vi "svx_Colormap Response User Shortcut Selection.vi"(6 "Action In":T4, 7 "Data In":T3 {"Y scale"."multiplier" format="%.2f"; "Y scale"."offset" format="%.2f"; "X scale"."multiplier" format="%.2f"; "X scale"."offset" format="%.2f"; "spectral map" format="%.2f"}, 8 "Color Map in":refnum<vi>, 9 "Refnum":refnum<vi>, 10 "ItemTag":string, 11 "State in":T1={"RefQueue"=refnum, "Properties/Undo"=refnum, "Bound"={"Width"=0, "Height"=0}, "Plot Area:Colors"={"FG Color"=11776947, "BG Color"=0}, "scale legend visible?"=FALSE, "graph palette visible?"=FALSE, "cursor palette visible?"=FALSE, "Ignore Array"=TRUE, "Smooth Update"=FALSE, "Z Scale"={"Z Scale.Scale Fit"=2, "Z Scale.Name Label.Text"="Amplitude", "Z Scale.Interpolate Color"=TRUE, "Visible"=TRUE, "Label Visible"=TRUE, "format string"="%#.2g", "Z Scale.Range"={"Minimum"=0.0, "Maximum"=500.0}}, "X Scale"={"X Scale.Scale Fit"=2, "X Scale.Offset and Multiplier"={"Offset"=0.0, "Multiplier"=1.0}, "X Scale.Name Label.Text"="Time", "X Scale.Range"={"Minimum"=0.0, "Maximum"=10.0}, "Visible"=TRUE, "Label Visible"=TRUE, "format string"="%#.2g"}, "Y Scale"={"Y Scale.Scale Fit"=2, "Y Scale.Offset and Multiplier"={"Offset"=0.0, "Multiplier"=1.0}, "Y Scale.Name Label.Text"="Frequency", "Y Scale.Range"={"Minimum"=0.0, "Maximum"=500.0}, "Visible"=TRUE, "Label Visible"=TRUE, "format string"="%#.2g"}, "Annotation List"=[], "Cursor List"=[], "Display Frequency Lines"=TRUE, "Display Order Lines"=TRUE, "Display Order text"=TRUE, "Display Frequency text"=TRUE, "Order Lineproperty"={"Line"={"Width"=1, "Style"=enum."Dash"}, "color"=0}, "Order Textproperty"={"Test size"=11, "color"=16777222, "background"=16777216}, "Orders"=[], "Frequency"=[], "Frequency Lineproperty"={"Line"={"Width"=1, "Style"=enum."Dash"}, "color"=0}, "Frequency Textproperty"={"Test size"=11, "color"=16777222, "background"=16777216}, "Display Order from Cursor"=FALSE, "Display Freq from Cursor"=FALSE, "Active Cursor"=0, "Selected Cursors"=[], "Cursor Move"=refnum, "Scale Range Change"=refnum}) -> (0 "Events":T2[](array[typedef]), 3 "State out":T1={"RefQueue"=refnum, "Properties/Undo"=refnum, "Bound"={"Width"=0, "Height"=0}, "Plot Area:Colors"={"FG Color"=11776947, "BG Color"=0}, "scale legend visible?"=FALSE, "graph palette visible?"=FALSE, "cursor palette visible?"=FALSE, "Ignore Array"=TRUE, "Smooth Update"=FALSE, "Z Scale"={"Z Scale.Scale Fit"=2, "Z Scale.Name Label.Text"="Amplitude", "Z Scale.Interpolate Color"=TRUE, "Visible"=TRUE, "Label Visible"=TRUE, "format string"="%#.2g", "Z Scale.Range"={"Minimum"=0.0, "Maximum"=500.0}}, "X Scale"={"X Scale.Scale Fit"=2, "X Scale.Offset and Multiplier"={"Offset"=0.0, "Multiplier"=1.0}, "X Scale.Name Label.Text"="Time", "X Scale.Range"={"Minimum"=0.0, "Maximum"=10.0}, "Visible"=TRUE, "Label Visible"=TRUE, "format string"="%#.2g"}, "Y Scale"={"Y Scale.Scale Fit"=2, "Y Scale.Offset and Multiplier"={"Offset"=0.0, "Multiplier"=1.0}, "Y Scale.Name Label.Text"="Frequency", "Y Scale.Range"={"Minimum"=0.0, "Maximum"=500.0}, "Visible"=TRUE, "Label Visible"=TRUE, "format string"="%#.2g"}, "Annotation List"=[], "Cursor List"=[], "Display Frequency Lines"=TRUE, "Display Order Lines"=TRUE, "Display Order text"=TRUE, "Display Frequency text"=TRUE, "Order Lineproperty"={"Line"={"Width"=1, "Style"=enum."Dash"}, "color"=0}, "Order Textproperty"={"Test size"=11, "color"=16777222, "background"=16777216}, "Orders"=[], "Frequency"=[], "Frequency Lineproperty"={"Line"={"Width"=1, "Style"=enum."Dash"}, "color"=0}, "Frequency Textproperty"={"Test size"=11, "color"=16777222, "background"=16777216}, "Display Order from Cursor"=FALSE, "Display Freq from Cursor"=FALSE, "Active Cursor"=0, "Selected Cursors"=[], "Cursor Move"=refnum, "Scale Range Change"=refnum}, 4 "Action":T4)   [LabVIEW 2017, in "SVX Colormap.xctl"]
uses:
  <vilib>/addons/_XControls/Colormap/SVX Colormap.xctl
  <vilib>/_xctls/Action.ctl
  <vilib>/addons/_XControls/Colormap/subVIs/svx_Colormap Data.ctl
  <vilib>/addons/_XControls/Colormap/TypeDef/svx_Colormap_Event.ctl
  <vilib>/addons/_XControls/Colormap/subVIs/svx_Colormap State.ctl
  <vilib>/addons/_XControls/Colormap/TypeDef/svx_Colormap_InnerState.ctl
  <vilib>/_xctls/XControlSupport.lvlib
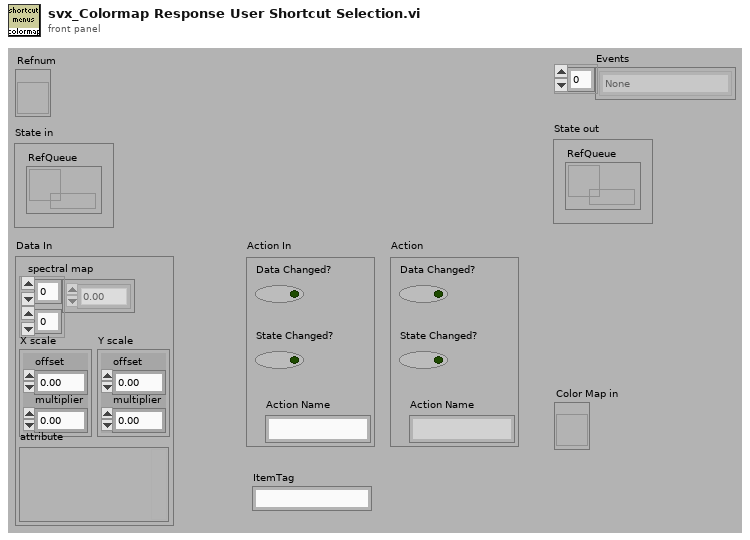
[diagram p1: front panel]
types:
  T1 = typedef "SVX Colormap.xctl/svx_Colormap State.ctl" = cluster{"RefQueue":refnum<queue>, "Properties/Undo":refnum<queue>, "Bound":cluster{"Width":u32, "Height":u32}, "Plot Area:Colors":cluster{"FG Color":u32, "BG Color":u32}, "scale legend visible?":bool, "graph palette visible?":bool, "cursor palette visible?":bool, "Ignore Array":bool, "Smooth Update":bool, "Z Scale":cluster{"Z Scale.Scale Fit":u8, "Z Scale.Name Label.Text":string, "Z Scale.Interpolate Color":bool, "Visible":bool, "Label Visible":bool, "format string":string, "Z Scale.Range":cluster{"Minimum":dbl, "Maximum":dbl}}, "X Scale":cluster{"X Scale.Scale Fit":u8, "X Scale.Offset and Multiplier":cluster{"Offset":dbl, "Multiplier":dbl}, "X Scale.Name Label.Text":string, "X Scale.Range":cluster{"Minimum":dbl, "Maximum":dbl}, "Visible":bool, "Label Visible":bool, "format string":string}, "Y Scale":cluster{"Y Scale.Scale Fit":u8, "Y Scale.Offset and Multiplier":cluster{"Offset":dbl, "Multiplier":dbl}, "Y Scale.Name Label.Text":string, "Y Scale.Range":cluster{"Minimum":dbl, "Maximum":dbl}, "Visible":bool, "Label Visible":bool, "format string":string}, "Annotation List":cluster{"Name":string, "Color":u32, "Style":u8, "Point Style":u8, "Name Visible":bool, "Allow Drag":bool, "Annotation Mode":u32, "Plot":i32, "Index":i32, "Position":cluster{"X":dbl, "Y":dbl}, "X Scale":u32, "Y Scale":u32, "Show Arrow":bool, "Lock Name":bool, "Plot Area":i32, "Label Offset":cluster{"X":dbl, "Y":dbl}}[], "Cursor List":cluster{"Name":string, "Color":u32, "Style":u8, "Point Style":u8, "Name Visible":bool, "Allow Drag":bool, "Cursor Mode":u32, "Plot":i32, "Index":i32, "Position":cluster{"X":dbl, "Y":dbl}, "X Scale":u32, "Y Scale":u32, "Watch Plots":i32[], "Watch All Plots":bool, "Plot Area":i32, "Label Offset":cluster{"X":dbl, "Y":dbl}}[], "Display Frequency Lines":bool, "Display Order Lines":bool, "Display Order text":bool, "Display Frequency text":bool, "Order Lineproperty":cluster{"Line":cluster{"Width":u16, "Style":enum32{"Solid", "Dash", "Dot", "DashDot", "DashDotDot"}}, "color":u32}, "Order Textproperty":cluster{"Test size":i16, "color":u32, "background":u32}, "Orders":dbl[], "Frequency":dbl[], "Frequency Lineproperty":cluster{"Line":cluster{"Width":u16, "Style":enum32{"Solid", "Dash", "Dot", "DashDot", "DashDotDot"}}, "color":u32}, "Frequency Textproperty":cluster{"Test size":i16, "color":u32, "background":u32}, "Display Order from Cursor":bool, "Display Freq from Cursor":bool, "Active Cursor":u32, "Selected Cursors":u32[], "Cursor Move":refnum<user-event>, "Scale Range Change":refnum<user-event>}
  T2 = typedef "SVX Colormap.xctl/svx_Colormap_Event.ctl" = enum16{"None", "[Axis] X Range", "[Axis] Y Range", "[Axis] Z Range", "[Axis] Range", "[Axis] X FString", "[Axis] Y FString", "[Axis] Z FString", "[Axis] X Name", "[Axis] X ScaleVis", "[Axis] X NameVis", "[Axis] Y Name", "[Axis] Y ScaleVis", "[Axis] Y NameVis", "[Axis] Z Name", "[Axis] Z ScaleVis", "[Axis] Z NameVis", "[Image] Line", "[Axis] Z Interp", "[Data] Update", "[Layout] Resize", "[ColorTable] Ignore Array", "[Legend] ScaleVis", "[Legend] GPVis", "[Legend] CPVis", "[Smooth] Update", "[Cursor] Update", "[Plot Area] Colors", "[Size] Minimum", "[Annotation] Update", "[Properties Dialog]", "[Axis] Autoscale X", "[Axis] Autoscale Y", "[Axis] Autoscale Z"}
  T3 = typedef "SVX Colormap.xctl/svx_Colormap Data.ctl" = cluster{"spectral map":dbl[][], "X scale":cluster{"offset":dbl, "multiplier":dbl}, "Y scale":cluster{"offset":dbl, "multiplier":dbl}, "attribute":variant}
  T4 = typedef "XControlSupport.lvlib/Action.ctl" = cluster{"Data Changed?":bool, "State Changed?":bool, "Action Name":string}
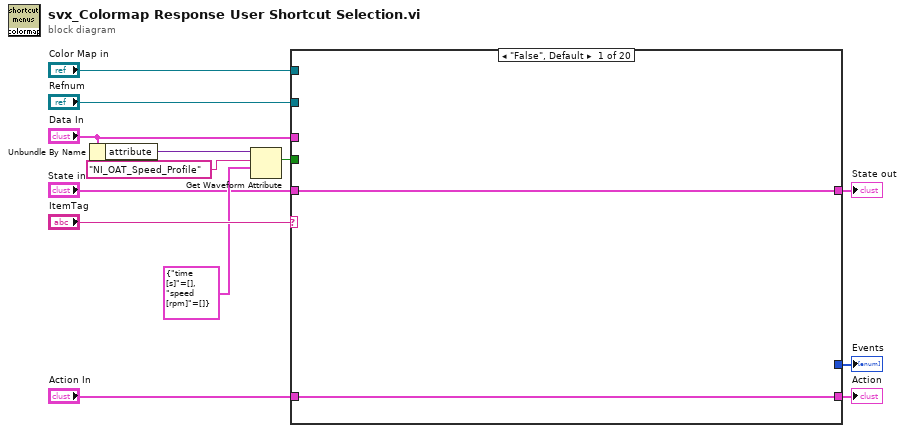
[diagram p0: block diagram]
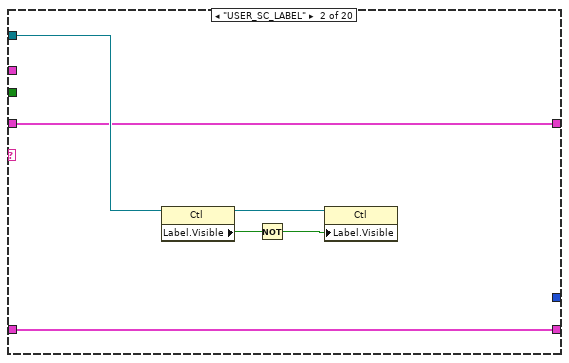
[diagram p2: hidden frame]
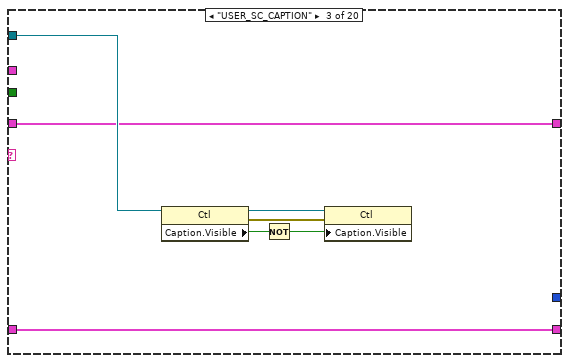
[diagram p3: hidden frame]
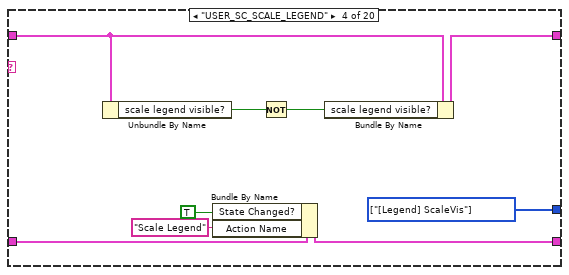
[diagram p4: hidden frame]
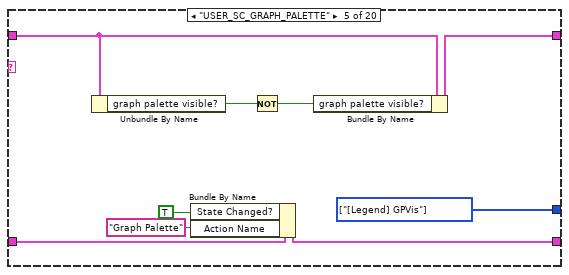
[diagram p5: hidden frame]
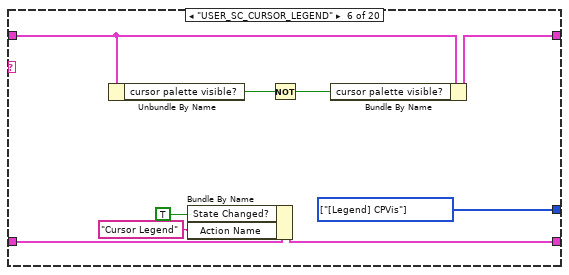
[diagram p6: hidden frame]
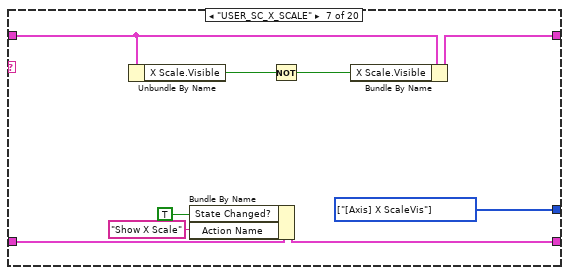
[diagram p7: hidden frame]
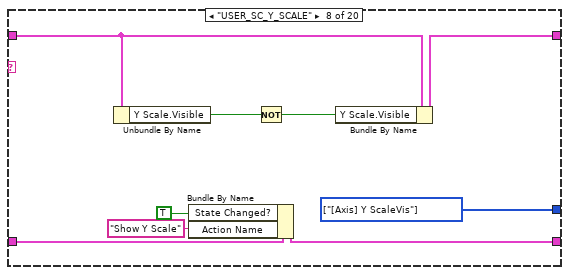
[diagram p8: hidden frame]
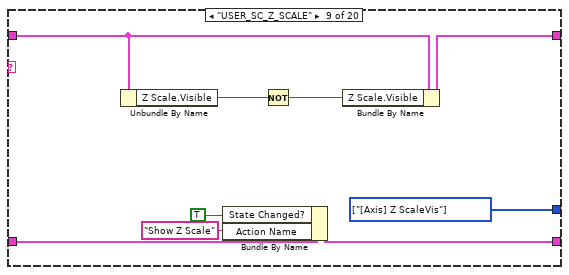
[diagram p9: hidden frame]
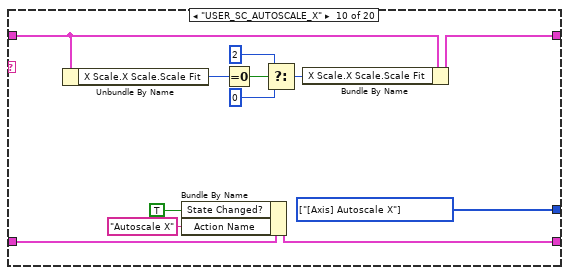
[diagram p10: hidden frame]
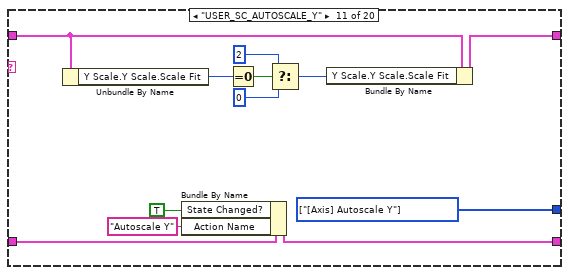
[diagram p11: hidden frame]
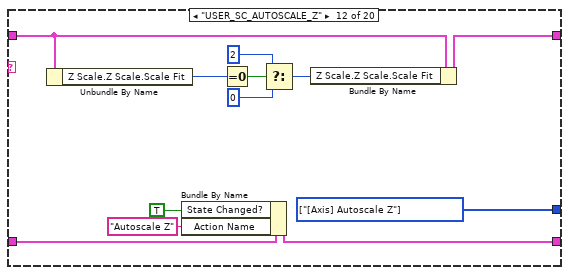
[diagram p12: hidden frame]
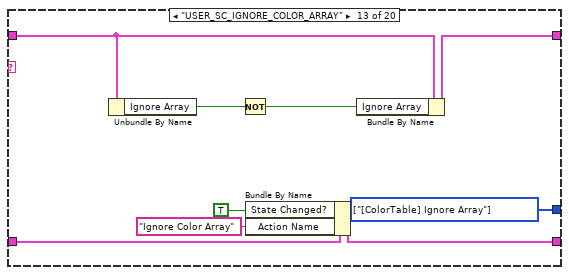
[diagram p13: hidden frame]
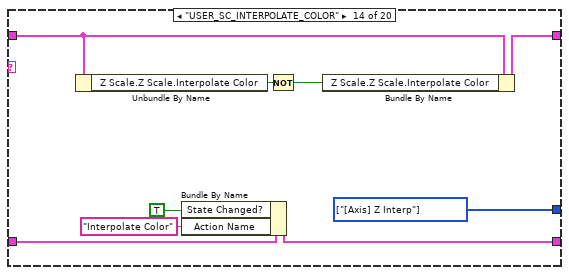
[diagram p14: hidden frame]
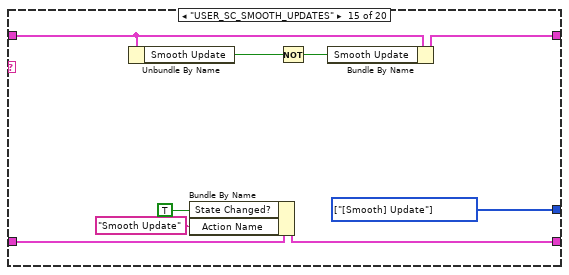
[diagram p15: hidden frame]
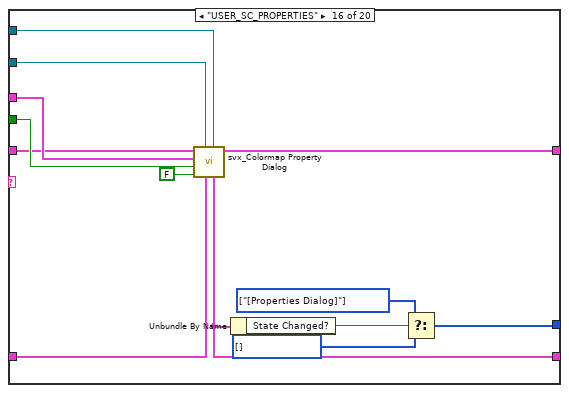
[diagram p16: hidden frame]
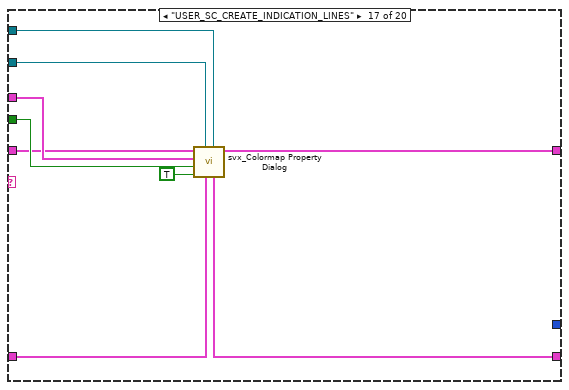
[diagram p17: hidden frame]
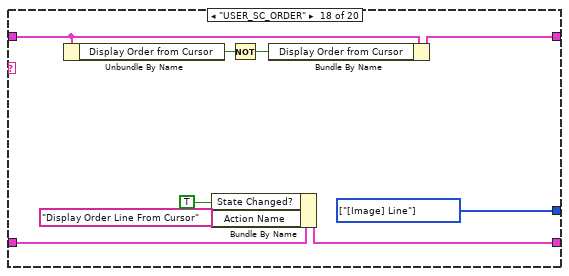
[diagram p18: hidden frame]
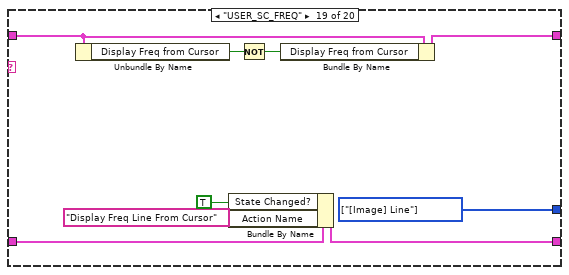
[diagram p19: hidden frame]
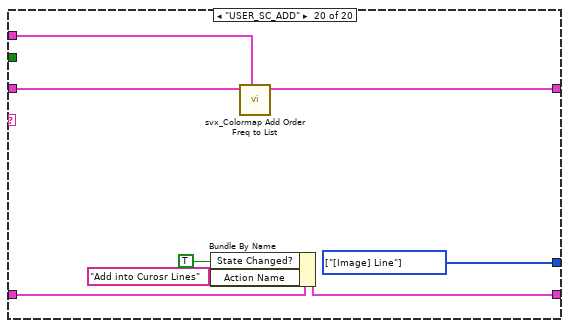
[diagram p20: hidden frame]
diagram:
  n1 = Unbundle By Name("Data In") -> ("attribute"=w9:variant)
  n2 = Get Waveform Attribute(5:cluster{"time [s]":dbl[], "speed [rpm]":dbl[]} {"time [s]"=[], "speed [rpm]"=[]} ("speed profile"), 6:"NI_OAT_Speed_Profile" ("name"), 7:w9) -> (2:w6:bool)  [unwired: 1 in, 3 out]
  n3 = case shown="\"False\", Default" "ItemTag" {
    tunnel: "Refnum" -> [_ w18 w24 _ _ _ _ _ _ _ _ _ _ _ _ w156 w164 _ _ _]
    tunnel: "Action In" -> [w15 w16 w22 w37 w46 w55 w62 w71 w80 w94 w106 w118 w127 w136 w145 w158 w166 w171 w178 w190]
    tunnel: [w15 w16 w22 w36 w45 w54 w61 w70 w79 w93 w105 w117 w126 w135 w144 w150 w167 w170 w179 w189] -> w11
    tunnel: "Color Map in" -> [_ _ _ _ _ _ _ _ _ _ _ _ _ _ _ w155 w163 _ _ _]
    tunnel: "State in" -> [w14 w17 w23 w31 w40 w49 w58 w67 w76 w89 w101 w113 w121 w131 w139 w152 w160 w176 w181 w191]
    tunnel: [w14 w17 w23 w33 w39 w48 w57 w66 w75 w90 w102 w114 w120 w132 w141 w157 w165 w175 w180 w193] -> w1
    tunnel: [_ _ _ w32 w38 w47 w56 w65 w74 w88 w100 w112 w119 w128 w137 w148 _ w168 w177 w186] -> w3
    tunnel: w6 -> [_ _ _ _ _ _ _ _ _ _ _ _ _ _ _ w153 w161 _ _ _]
    tunnel: "Data In" -> [_ _ _ _ _ _ _ _ _ _ _ _ _ _ _ w154 w162 _ _ w192]
    frame "False", Default {
    }
    frame "USER_SC_LABEL" {
      n4 = property class="Ctl"(reference=w18) -> (reference out=w21:refnum<vi>, "Label.Visible"=w20:bool)  [unwired: 1 in, 1 out]
      n5 = Not(x=w20) -> (.not. x?=w19:bool)
      n6 = property class="Ctl"(reference=w21, "Label.Visible"=w19) -> ()  [unwired: 1 in, 2 out]
    }
    frame "USER_SC_CAPTION" {
      n7 = property class="Ctl"(reference=w24) -> (reference out=w28:refnum<vi>, error out=w27:errorcluster, "Caption.Visible"=w26:bool)  [unwired: 1 in]
      n8 = Not(x=w26) -> (.not. x?=w25:bool)
      n9 = property class="Ctl"(reference=w28, error in=w27, "Caption.Visible"=w25) -> ()  [unwired: 2 out]
    }
    frame "USER_SC_SCALE_LEGEND" {
      w32 = T2[] [enum."[Legend] ScaleVis"] items=["None", "[Axis] X Range", "[Axis] Y Range", "[Axis] Z Range", "[Axis] Range", "[Axis] X FString", "[Axis] Y FString", "[Axis] Z FString", "[Axis] X Name", "[Axis] X ScaleVis", "[Axis] X NameVis", "[Axis] Y Name", "[Axis] Y ScaleVis", "[Axis] Y NameVis", "[Axis] Z Name", "[Axis] Z ScaleVis", "[Axis] Z NameVis", "[Image] Line", "[Axis] Z Interp", "[Data] Update", "[Layout] Resize", "[ColorTable] Ignore Array", "[Legend] ScaleVis", "[Legend] GPVis", "[Legend] CPVis", "[Smooth] Update", "[Cursor] Update", "[Plot Area] Colors", "[Size] Minimum", "[Annotation] Update", "[Properties Dialog]", "[Axis] Autoscale X", "[Axis] Autoscale Y", "[Axis] Autoscale Z"]
      n10 = Unbundle By Name(w31) -> ("scale legend visible?"=w30:bool)
      n11 = Bundle By Name(cluster=w37, "State Changed?"=TRUE, "Action Name"="Scale Legend") -> (w36:T4)
      n12 = Not(x=w30) -> (.not. x?=w29:bool)
      n13 = Bundle By Name(cluster=w31, "scale legend visible?"=w29) -> (w33:T1)
    }
    frame "USER_SC_GRAPH_PALETTE" {
      w38 = T2[] [enum."[Legend] GPVis"] items=["None", "[Axis] X Range", "[Axis] Y Range", "[Axis] Z Range", "[Axis] Range", "[Axis] X FString", "[Axis] Y FString", "[Axis] Z FString", "[Axis] X Name", "[Axis] X ScaleVis", "[Axis] X NameVis", "[Axis] Y Name", "[Axis] Y ScaleVis", "[Axis] Y NameVis", "[Axis] Z Name", "[Axis] Z ScaleVis", "[Axis] Z NameVis", "[Image] Line", "[Axis] Z Interp", "[Data] Update", "[Layout] Resize", "[ColorTable] Ignore Array", "[Legend] ScaleVis", "[Legend] GPVis", "[Legend] CPVis", "[Smooth] Update", "[Cursor] Update", "[Plot Area] Colors", "[Size] Minimum", "[Annotation] Update", "[Properties Dialog]", "[Axis] Autoscale X", "[Axis] Autoscale Y", "[Axis] Autoscale Z"]
      n14 = Unbundle By Name(w40) -> ("graph palette visible?"=w42:bool)
      n15 = Bundle By Name(cluster=w46, "State Changed?"=TRUE, "Action Name"="Graph Palette") -> (w45:T4)
      n16 = Not(x=w42) -> (.not. x?=w41:bool)
      n17 = Bundle By Name(cluster=w40, "graph palette visible?"=w41) -> (w39:T1)
    }
    frame "USER_SC_CURSOR_LEGEND" {
      w47 = T2[] [enum."[Legend] CPVis"] items=["None", "[Axis] X Range", "[Axis] Y Range", "[Axis] Z Range", "[Axis] Range", "[Axis] X FString", "[Axis] Y FString", "[Axis] Z FString", "[Axis] X Name", "[Axis] X ScaleVis", "[Axis] X NameVis", "[Axis] Y Name", "[Axis] Y ScaleVis", "[Axis] Y NameVis", "[Axis] Z Name", "[Axis] Z ScaleVis", "[Axis] Z NameVis", "[Image] Line", "[Axis] Z Interp", "[Data] Update", "[Layout] Resize", "[ColorTable] Ignore Array", "[Legend] ScaleVis", "[Legend] GPVis", "[Legend] CPVis", "[Smooth] Update", "[Cursor] Update", "[Plot Area] Colors", "[Size] Minimum", "[Annotation] Update", "[Properties Dialog]", "[Axis] Autoscale X", "[Axis] Autoscale Y", "[Axis] Autoscale Z"]
      n18 = Unbundle By Name(w49) -> ("cursor palette visible?"=w51:bool)
      n19 = Bundle By Name(cluster=w55, "State Changed?"=TRUE, "Action Name"="Cursor Legend") -> (w54:T4)
      n20 = Not(x=w51) -> (.not. x?=w50:bool)
      n21 = Bundle By Name(cluster=w49, "cursor palette visible?"=w50) -> (w48:T1)
    }
    frame "USER_SC_X_SCALE" {
      w56 = T2[] [enum."[Axis] X ScaleVis"] items=["None", "[Axis] X Range", "[Axis] Y Range", "[Axis] Z Range", "[Axis] Range", "[Axis] X FString", "[Axis] Y FString", "[Axis] Z FString", "[Axis] X Name", "[Axis] X ScaleVis", "[Axis] X NameVis", "[Axis] Y Name", "[Axis] Y ScaleVis", "[Axis] Y NameVis", "[Axis] Z Name", "[Axis] Z ScaleVis", "[Axis] Z NameVis", "[Image] Line", "[Axis] Z Interp", "[Data] Update", "[Layout] Resize", "[ColorTable] Ignore Array", "[Legend] ScaleVis", "[Legend] GPVis", "[Legend] CPVis", "[Smooth] Update", "[Cursor] Update", "[Plot Area] Colors", "[Size] Minimum", "[Annotation] Update", "[Properties Dialog]", "[Axis] Autoscale X", "[Axis] Autoscale Y", "[Axis] Autoscale Z"]
      n22 = Unbundle By Name(w58) -> ("X Scale.Visible"=w60:bool)
      n23 = Bundle By Name(cluster=w62, "State Changed?"=TRUE, "Action Name"="Show X Scale") -> (w61:T4)
      n24 = Not(x=w60) -> (.not. x?=w59:bool)
      n25 = Bundle By Name(cluster=w58, "X Scale.Visible"=w59) -> (w57:T1)
    }
    frame "USER_SC_Y_SCALE" {
      w65 = T2[] [enum."[Axis] Y ScaleVis"] items=["None", "[Axis] X Range", "[Axis] Y Range", "[Axis] Z Range", "[Axis] Range", "[Axis] X FString", "[Axis] Y FString", "[Axis] Z FString", "[Axis] X Name", "[Axis] X ScaleVis", "[Axis] X NameVis", "[Axis] Y Name", "[Axis] Y ScaleVis", "[Axis] Y NameVis", "[Axis] Z Name", "[Axis] Z ScaleVis", "[Axis] Z NameVis", "[Image] Line", "[Axis] Z Interp", "[Data] Update", "[Layout] Resize", "[ColorTable] Ignore Array", "[Legend] ScaleVis", "[Legend] GPVis", "[Legend] CPVis", "[Smooth] Update", "[Cursor] Update", "[Plot Area] Colors", "[Size] Minimum", "[Annotation] Update", "[Properties Dialog]", "[Axis] Autoscale X", "[Axis] Autoscale Y", "[Axis] Autoscale Z"]
      n26 = Unbundle By Name(w67) -> ("Y Scale.Visible"=w69:bool)
      n27 = Bundle By Name(cluster=w71, "State Changed?"=TRUE, "Action Name"="Show Y Scale") -> (w70:T4)
      n28 = Not(x=w69) -> (.not. x?=w68:bool)
      n29 = Bundle By Name(cluster=w67, "Y Scale.Visible"=w68) -> (w66:T1)
    }
    frame "USER_SC_Z_SCALE" {
      w74 = T2[] [enum."[Axis] Z ScaleVis"] items=["None", "[Axis] X Range", "[Axis] Y Range", "[Axis] Z Range", "[Axis] Range", "[Axis] X FString", "[Axis] Y FString", "[Axis] Z FString", "[Axis] X Name", "[Axis] X ScaleVis", "[Axis] X NameVis", "[Axis] Y Name", "[Axis] Y ScaleVis", "[Axis] Y NameVis", "[Axis] Z Name", "[Axis] Z ScaleVis", "[Axis] Z NameVis", "[Image] Line", "[Axis] Z Interp", "[Data] Update", "[Layout] Resize", "[ColorTable] Ignore Array", "[Legend] ScaleVis", "[Legend] GPVis", "[Legend] CPVis", "[Smooth] Update", "[Cursor] Update", "[Plot Area] Colors", "[Size] Minimum", "[Annotation] Update", "[Properties Dialog]", "[Axis] Autoscale X", "[Axis] Autoscale Y", "[Axis] Autoscale Z"]
      n30 = Unbundle By Name(w76) -> ("Z Scale.Visible"=w78:bool)
      n31 = Bundle By Name(cluster=w80, "State Changed?"=TRUE, "Action Name"="Show Z Scale") -> (w79:T4)
      n32 = Not(x=w78) -> (.not. x?=w77:bool)
      n33 = Bundle By Name(cluster=w76, "Z Scale.Visible"=w77) -> (w75:T1)
    }
    frame "USER_SC_AUTOSCALE_X" {
      w88 = T2[] [enum."[Axis] Autoscale X"] items=["None", "[Axis] X Range", "[Axis] Y Range", "[Axis] Z Range", "[Axis] Range", "[Axis] X FString", "[Axis] Y FString", "[Axis] Z FString", "[Axis] X Name", "[Axis] X ScaleVis", "[Axis] X NameVis", "[Axis] Y Name", "[Axis] Y ScaleVis", "[Axis] Y NameVis", "[Axis] Z Name", "[Axis] Z ScaleVis", "[Axis] Z NameVis", "[Image] Line", "[Axis] Z Interp", "[Data] Update", "[Layout] Resize", "[ColorTable] Ignore Array", "[Legend] ScaleVis", "[Legend] GPVis", "[Legend] CPVis", "[Smooth] Update", "[Cursor] Update", "[Plot Area] Colors", "[Size] Minimum", "[Annotation] Update", "[Properties Dialog]", "[Axis] Autoscale X", "[Axis] Autoscale Y", "[Axis] Autoscale Z"]
      n34 = Unbundle By Name(w89) -> ("X Scale.X Scale.Scale Fit"=w87:u8)
      n35 = Bundle By Name(cluster=w94, "State Changed?"=TRUE, "Action Name"="Autoscale X") -> (w93:T4)
      n36 = Equal To 0?(x=w87) -> (x = 0?=w86:bool)
      n37 = Select(t=u8 2 ("X Scale.X Scale.Scale Fit"), s=w86, f=u8 0 ("X Scale.X Scale.Scale Fit")) -> (s? t:f=w83:u8)
      n38 = Bundle By Name(cluster=w89, "X Scale.X Scale.Scale Fit"=w83) -> (w90:T1)
    }
    frame "USER_SC_AUTOSCALE_Y" {
      w100 = T2[] [enum."[Axis] Autoscale Y"] items=["None", "[Axis] X Range", "[Axis] Y Range", "[Axis] Z Range", "[Axis] Range", "[Axis] X FString", "[Axis] Y FString", "[Axis] Z FString", "[Axis] X Name", "[Axis] X ScaleVis", "[Axis] X NameVis", "[Axis] Y Name", "[Axis] Y ScaleVis", "[Axis] Y NameVis", "[Axis] Z Name", "[Axis] Z ScaleVis", "[Axis] Z NameVis", "[Image] Line", "[Axis] Z Interp", "[Data] Update", "[Layout] Resize", "[ColorTable] Ignore Array", "[Legend] ScaleVis", "[Legend] GPVis", "[Legend] CPVis", "[Smooth] Update", "[Cursor] Update", "[Plot Area] Colors", "[Size] Minimum", "[Annotation] Update", "[Properties Dialog]", "[Axis] Autoscale X", "[Axis] Autoscale Y", "[Axis] Autoscale Z"]
      n39 = Unbundle By Name(w101) -> ("Y Scale.Y Scale.Scale Fit"=w96:u8)
      n40 = Bundle By Name(cluster=w106, "State Changed?"=TRUE, "Action Name"="Autoscale Y") -> (w105:T4)
      n41 = Equal To 0?(x=w96) -> (x = 0?=w99:bool)
      n42 = Select(t=u8 2 ("X Scale.X Scale.Scale Fit"), s=w99, f=u8 0 ("X Scale.X Scale.Scale Fit")) -> (s? t:f=w95:u8)
      n43 = Bundle By Name(cluster=w101, "Y Scale.Y Scale.Scale Fit"=w95) -> (w102:T1)
    }
    frame "USER_SC_AUTOSCALE_Z" {
      w112 = T2[] [enum."[Axis] Autoscale Z"] items=["None", "[Axis] X Range", "[Axis] Y Range", "[Axis] Z Range", "[Axis] Range", "[Axis] X FString", "[Axis] Y FString", "[Axis] Z FString", "[Axis] X Name", "[Axis] X ScaleVis", "[Axis] X NameVis", "[Axis] Y Name", "[Axis] Y ScaleVis", "[Axis] Y NameVis", "[Axis] Z Name", "[Axis] Z ScaleVis", "[Axis] Z NameVis", "[Image] Line", "[Axis] Z Interp", "[Data] Update", "[Layout] Resize", "[ColorTable] Ignore Array", "[Legend] ScaleVis", "[Legend] GPVis", "[Legend] CPVis", "[Smooth] Update", "[Cursor] Update", "[Plot Area] Colors", "[Size] Minimum", "[Annotation] Update", "[Properties Dialog]", "[Axis] Autoscale X", "[Axis] Autoscale Y", "[Axis] Autoscale Z"]
      n44 = Unbundle By Name(w113) -> ("Z Scale.Z Scale.Scale Fit"=w108:u8)
      n45 = Bundle By Name(cluster=w118, "State Changed?"=TRUE, "Action Name"="Autoscale Z") -> (w117:T4)
      n46 = Equal To 0?(x=w108) -> (x = 0?=w111:bool)
      n47 = Select(t=u8 2 ("X Scale.X Scale.Scale Fit"), s=w111, f=u8 0 ("X Scale.X Scale.Scale Fit")) -> (s? t:f=w107:u8)
      n48 = Bundle By Name(cluster=w113, "Z Scale.Z Scale.Scale Fit"=w107) -> (w114:T1)
    }
    frame "USER_SC_IGNORE_COLOR_ARRAY" {
      w119 = T2[] [enum."[ColorTable] Ignore Array"] items=["None", "[Axis] X Range", "[Axis] Y Range", "[Axis] Z Range", "[Axis] Range", "[Axis] X FString", "[Axis] Y FString", "[Axis] Z FString", "[Axis] X Name", "[Axis] X ScaleVis", "[Axis] X NameVis", "[Axis] Y Name", "[Axis] Y ScaleVis", "[Axis] Y NameVis", "[Axis] Z Name", "[Axis] Z ScaleVis", "[Axis] Z NameVis", "[Image] Line", "[Axis] Z Interp", "[Data] Update", "[Layout] Resize", "[ColorTable] Ignore Array", "[Legend] ScaleVis", "[Legend] GPVis", "[Legend] CPVis", "[Smooth] Update", "[Cursor] Update", "[Plot Area] Colors", "[Size] Minimum", "[Annotation] Update", "[Properties Dialog]", "[Axis] Autoscale X", "[Axis] Autoscale Y", "[Axis] Autoscale Z"]
      n49 = Unbundle By Name(w121) -> ("Ignore Array"=w123:bool)
      n50 = Not(x=w123) -> (.not. x?=w122:bool)
      n51 = Bundle By Name(cluster=w127, "State Changed?"=TRUE, "Action Name"="Ignore Color Array") -> (w126:T4)
      n52 = Bundle By Name(cluster=w121, "Ignore Array"=w122) -> (w120:T1)
    }
    frame "USER_SC_INTERPOLATE_COLOR" {
      w128 = T2[] [enum."[Axis] Z Interp"] items=["None", "[Axis] X Range", "[Axis] Y Range", "[Axis] Z Range", "[Axis] Range", "[Axis] X FString", "[Axis] Y FString", "[Axis] Z FString", "[Axis] X Name", "[Axis] X ScaleVis", "[Axis] X NameVis", "[Axis] Y Name", "[Axis] Y ScaleVis", "[Axis] Y NameVis", "[Axis] Z Name", "[Axis] Z ScaleVis", "[Axis] Z NameVis", "[Image] Line", "[Axis] Z Interp", "[Data] Update", "[Layout] Resize", "[ColorTable] Ignore Array", "[Legend] ScaleVis", "[Legend] GPVis", "[Legend] CPVis", "[Smooth] Update", "[Cursor] Update", "[Plot Area] Colors", "[Size] Minimum", "[Annotation] Update", "[Properties Dialog]", "[Axis] Autoscale X", "[Axis] Autoscale Y", "[Axis] Autoscale Z"]
      n53 = Unbundle By Name(w131) -> ("Z Scale.Z Scale.Interpolate Color"=w130:bool)
      n54 = Bundle By Name(cluster=w136, "State Changed?"=TRUE, "Action Name"="Interpolate Color") -> (w135:T4)
      n55 = Not(x=w130) -> (.not. x?=w129:bool)
      n56 = Bundle By Name(cluster=w131, "Z Scale.Z Scale.Interpolate Color"=w129) -> (w132:T1)
    }
    frame "USER_SC_SMOOTH_UPDATES" {
      w137 = T2[] [enum."[Smooth] Update"] items=["None", "[Axis] X Range", "[Axis] Y Range", "[Axis] Z Range", "[Axis] Range", "[Axis] X FString", "[Axis] Y FString", "[Axis] Z FString", "[Axis] X Name", "[Axis] X ScaleVis", "[Axis] X NameVis", "[Axis] Y Name", "[Axis] Y ScaleVis", "[Axis] Y NameVis", "[Axis] Z Name", "[Axis] Z ScaleVis", "[Axis] Z NameVis", "[Image] Line", "[Axis] Z Interp", "[Data] Update", "[Layout] Resize", "[ColorTable] Ignore Array", "[Legend] ScaleVis", "[Legend] GPVis", "[Legend] CPVis", "[Smooth] Update", "[Cursor] Update", "[Plot Area] Colors", "[Size] Minimum", "[Annotation] Update", "[Properties Dialog]", "[Axis] Autoscale X", "[Axis] Autoscale Y", "[Axis] Autoscale Z"]
      n57 = Unbundle By Name(w139) -> ("Smooth Update"=w140:bool)
      n58 = Bundle By Name(cluster=w145, "State Changed?"=TRUE, "Action Name"="Smooth Update") -> (w144:T4)
      n59 = Not(x=w140) -> (.not. x?=w138:bool)
      n60 = Bundle By Name(cluster=w139, "Smooth Update"=w138) -> (w141:T1)
    }
    frame "USER_SC_PROPERTIES" {
      w146 = T2[] [] items=["None", "[Axis] X Range", "[Axis] Y Range", "[Axis] Z Range", "[Axis] Range", "[Axis] X FString", "[Axis] Y FString", "[Axis] Z FString", "[Axis] X Name", "[Axis] X ScaleVis", "[Axis] X NameVis", "[Axis] Y Name", "[Axis] Y ScaleVis", "[Axis] Y NameVis", "[Axis] Z Name", "[Axis] Z ScaleVis", "[Axis] Z NameVis", "[Image] Line", "[Axis] Z Interp", "[Data] Update", "[Layout] Resize", "[ColorTable] Ignore Array", "[Legend] ScaleVis", "[Legend] GPVis", "[Legend] CPVis", "[Smooth] Update", "[Cursor] Update", "[Plot Area] Colors", "[Size] Minimum", "[Annotation] Update", "[Properties Dialog]", "[Axis] Autoscale X", "[Axis] Autoscale Y", "[Axis] Autoscale Z"] ("f")
      w147 = T2[] [enum."[Properties Dialog]"] items=["None", "[Axis] X Range", "[Axis] Y Range", "[Axis] Z Range", "[Axis] Range", "[Axis] X FString", "[Axis] Y FString", "[Axis] Z FString", "[Axis] X Name", "[Axis] X ScaleVis", "[Axis] X NameVis", "[Axis] Y Name", "[Axis] Y ScaleVis", "[Axis] Y NameVis", "[Axis] Z Name", "[Axis] Z ScaleVis", "[Axis] Z NameVis", "[Image] Line", "[Axis] Z Interp", "[Data] Update", "[Layout] Resize", "[ColorTable] Ignore Array", "[Legend] ScaleVis", "[Legend] GPVis", "[Legend] CPVis", "[Smooth] Update", "[Cursor] Update", "[Plot Area] Colors", "[Size] Minimum", "[Annotation] Update", "[Properties Dialog]", "[Axis] Autoscale X", "[Axis] Autoscale Y", "[Axis] Autoscale Z"]
      n61 = call <vilib>:"svx_Colormap Property Dialog.vi"("Color Map in"=w155, "Action In"=w158, "Refnum"=w156, "Cursor Lines only?"=FALSE, "Found Speed"=w153, "Data In"=w154, "State in"=w152) -> ("State out"=w157:T1, "Action"=w150:T4)  [unwired: 3 in]
      n62 = Unbundle By Name(w150) -> ("State Changed?"=w149:bool)
      n63 = Select(t=w147, s=w149, f=w146) -> (s? t:f=w148:T2[])
    }
    frame "USER_SC_CREATE_INDICATION_LINES" {
      n64 = call <vilib>:"svx_Colormap Property Dialog.vi"("Color Map in"=w163, "Action In"=w166, "Refnum"=w164, "Cursor Lines only?"=TRUE, "Found Speed"=w161, "Data In"=w162, "State in"=w160) -> ("State out"=w165:T1, "Action"=w167:T4)  [unwired: 3 in]
    }
    frame "USER_SC_ORDER" {
      w168 = T2[] [enum."[Image] Line"] items=["None", "[Axis] X Range", "[Axis] Y Range", "[Axis] Z Range", "[Axis] Range", "[Axis] X FString", "[Axis] Y FString", "[Axis] Z FString", "[Axis] X Name", "[Axis] X ScaleVis", "[Axis] X NameVis", "[Axis] Y Name", "[Axis] Y ScaleVis", "[Axis] Y NameVis", "[Axis] Z Name", "[Axis] Z ScaleVis", "[Axis] Z NameVis", "[Image] Line", "[Axis] Z Interp", "[Data] Update", "[Layout] Resize", "[ColorTable] Ignore Array", "[Legend] ScaleVis", "[Legend] GPVis", "[Legend] CPVis", "[Smooth] Update", "[Cursor] Update", "[Plot Area] Colors", "[Size] Minimum", "[Annotation] Update", "[Properties Dialog]", "[Axis] Autoscale X", "[Axis] Autoscale Y", "[Axis] Autoscale Z"]
      n65 = Unbundle By Name(w176) -> ("Display Order from Cursor"=w174:bool)
      n66 = Bundle By Name(cluster=w171, "State Changed?"=TRUE, "Action Name"="Display Order Line From Cursor") -> (w170:T4)
      n67 = Not(x=w174) -> (.not. x?=w169:bool)
      n68 = Bundle By Name(cluster=w176, "Display Order from Cursor"=w169) -> (w175:T1)
    }
    frame "USER_SC_FREQ" {
      w177 = T2[] [enum."[Image] Line"] items=["None", "[Axis] X Range", "[Axis] Y Range", "[Axis] Z Range", "[Axis] Range", "[Axis] X FString", "[Axis] Y FString", "[Axis] Z FString", "[Axis] X Name", "[Axis] X ScaleVis", "[Axis] X NameVis", "[Axis] Y Name", "[Axis] Y ScaleVis", "[Axis] Y NameVis", "[Axis] Z Name", "[Axis] Z ScaleVis", "[Axis] Z NameVis", "[Image] Line", "[Axis] Z Interp", "[Data] Update", "[Layout] Resize", "[ColorTable] Ignore Array", "[Legend] ScaleVis", "[Legend] GPVis", "[Legend] CPVis", "[Smooth] Update", "[Cursor] Update", "[Plot Area] Colors", "[Size] Minimum", "[Annotation] Update", "[Properties Dialog]", "[Axis] Autoscale X", "[Axis] Autoscale Y", "[Axis] Autoscale Z"]
      n69 = Unbundle By Name(w181) -> ("Display Freq from Cursor"=w185:bool)
      n70 = Bundle By Name(cluster=w178, "State Changed?"=TRUE, "Action Name"="Display Freq Line From Cursor") -> (w179:T4)
      n71 = Not(x=w185) -> (.not. x?=w184:bool)
      n72 = Bundle By Name(cluster=w181, "Display Freq from Cursor"=w184) -> (w180:T1)
    }
    frame "USER_SC_ADD" {
      w186 = T2[] [enum."[Image] Line"] items=["None", "[Axis] X Range", "[Axis] Y Range", "[Axis] Z Range", "[Axis] Range", "[Axis] X FString", "[Axis] Y FString", "[Axis] Z FString", "[Axis] X Name", "[Axis] X ScaleVis", "[Axis] X NameVis", "[Axis] Y Name", "[Axis] Y ScaleVis", "[Axis] Y NameVis", "[Axis] Z Name", "[Axis] Z ScaleVis", "[Axis] Z NameVis", "[Image] Line", "[Axis] Z Interp", "[Data] Update", "[Layout] Resize", "[ColorTable] Ignore Array", "[Legend] ScaleVis", "[Legend] GPVis", "[Legend] CPVis", "[Smooth] Update", "[Cursor] Update", "[Plot Area] Colors", "[Size] Minimum", "[Annotation] Update", "[Properties Dialog]", "[Axis] Autoscale X", "[Axis] Autoscale Y", "[Axis] Autoscale Z"]
      n73 = Bundle By Name(cluster=w190, "State Changed?"=TRUE, "Action Name"="Add into Curosr Lines") -> (w189:T4)
      n74 = call <vilib>:"svx_Colormap Add Order Freq to List.vi"("Data In"=w192, "State in"=w191) -> ("State out"=w193:T1)  [unwired: 9 in]
    }
  }
  "Action" <- w11
  "Events" <- w3
  "State out" <- w1
